vi "decode_tcp_buf.vi"(8 "error in (no error)":errorcluster, 11 "data in":string) -> (0 "error out":errorcluster, 3 "Data out":i32[](array[numeric]) format="%12d")   [LabVIEW 2014]
panel:
  in  "Force second":bool
  in  "Force first":bool
  out "Use first slot?":bool
  out "Waveform Graph":i32[][](graph)
  out "Input data long":i32[][](array[numeric]) format="%12d"
  # "This is obsolete, and was to hack around a weird problem with the Raspberry Pi eval setup that (due to my not knowing how to configure Linux alsa, drivers, etc., both input channels are showing up interleaved as mono, with non-determinstic left/right order.  So we have to figure out which one has the signal and pick it out.  This would be impossible if both channels had signal."
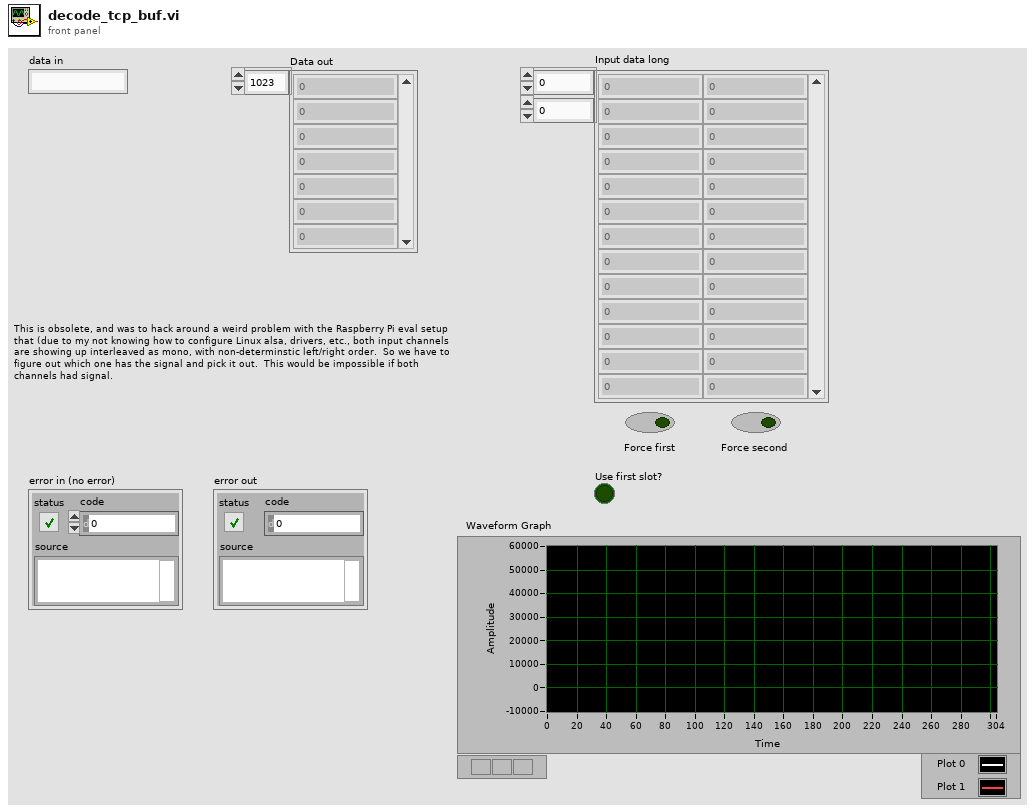
[diagram p1: front panel]
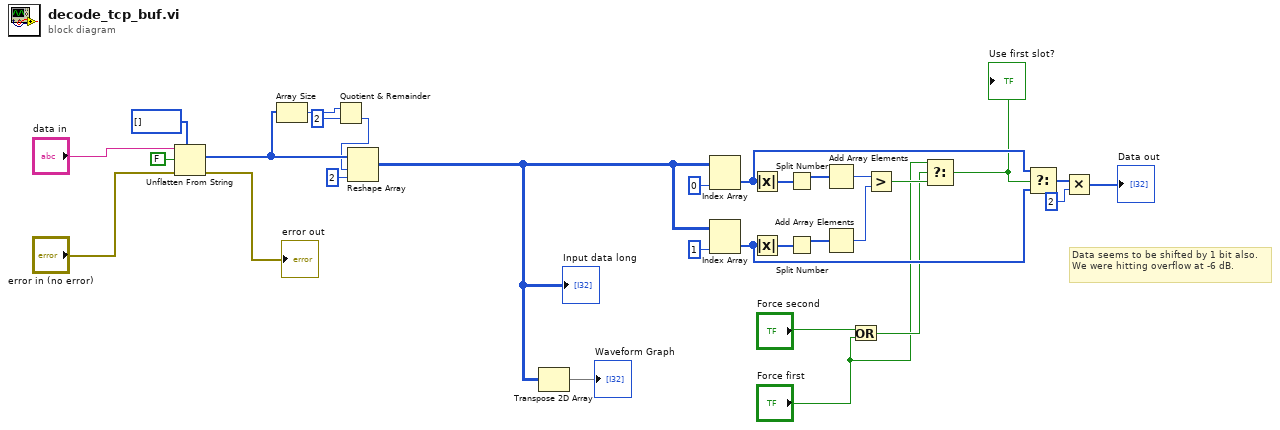
[diagram p0: block diagram]
diagram:
  # "Data seems to be shifted by 1 bit also.  We were hitting overflow at -6 dB."
  n1 = Unflatten From String(type=i32[] [], binary string="data in", data includes array or string size? (T)=FALSE, error in (no error)="error in (no error)") -> (value=w24:i32[], error out=→"error out":errorcluster)  [unwired: 1 in, 1 out]
  n2 = Array Size(array=w24) -> (size(s)=w23:i32)
  n3 = Quotient & Remainder(x=w23, y=2) -> (floor(x/y)=w21:i32)  [unwired: 1 out]
  n4 = Reshape Array(w24, w21, 2 ("dimension size")) -> (w9:i32[][])
  "Input data long" <- w9
  n5 = Transpose 2D Array(2D array=w9) -> (transposed array=→"Waveform Graph":i32[][])
  n6 = Index Array(array=w9, index (col)=0 ("disabled index (col)")) -> (element=w11:i32[])  [unwired: 1 in]
  n7 = Index Array(array=w9, index (col)=1 ("disabled index (col)")) -> (element=w10:i32[])  [unwired: 1 in]
  n8 = Absolute Value(x=w11) -> (abs(x)=w18:i32[])
  n9 = Absolute Value(x=w10) -> (abs(x)=w15:i32[])
  n10 = Split Number(x=w18) -> (hi(x)=w17:u16[])  [unwired: 1 out]
  n11 = Split Number(x=w15) -> (hi(x)=w16:u16[])  [unwired: 1 out]
  n12 = Add Array Elements(numeric array=w17) -> (sum=w13:u16)
  n13 = Add Array Elements(numeric array=w16) -> (sum=w12:u16)
  n14 = Or(x="Force second", y="Force first") -> (x .or. y?=w3:bool)
  n15 = Greater?(x=w13, y=w12) -> (0:w4:bool)
  n16 = Select(t="Force first", s=w3, f=w4) -> (s? t:f=w1:bool)
  "Use first slot?" <- w1
  n17 = Select(t=w11, s=w1, f=w10) -> (s? t:f=w8:i32[])
  n18 = Multiply(x=w8, y=2 ("sum")) -> (x*y=→"Data out":i32[])
